vi "ClimbWeightHandler.vi"(8 "error in (no error)":errorcluster, 10 "cClimbWeight":bool, 11 "MainQueue":refnum<queue>) -> (0 "error out":errorcluster)   [LabVIEW 2013]
uses:
  QueueInstruction.ctl
  SubsystemEnum.ctl
  ActionEnum.ctl
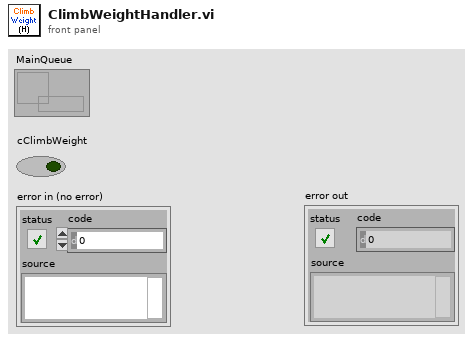
[diagram p1: front panel]
types:
  T1 = typedef "SubsystemEnum.ctl" = enum16{"TankDrive", "FirePneumatic", "Climber", "ClimbWeight", "ShooterAngle"}
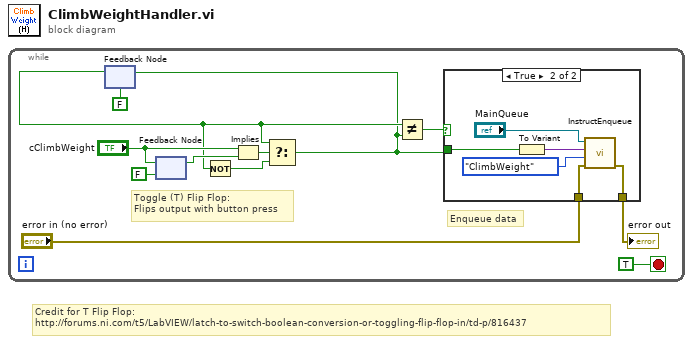
[diagram p0: block diagram]
diagram:
  # "Credit for T Flip Flop:\nhttp://forums.ni.com/t5/LabVIEW/latch-to-switch-boolean-conversion-or-toggling-flip-flop-in/td-p/816437"
  n1 = while {
    stop <- TRUE stop-if-true
    # "Enqueue data"
    # "Toggle (T) Flip Flop:\nFlips output with button press"
    n2 = feedback #1(FALSE) -> (w4:bool)
    n3 = feedback #2(FALSE ("cClimbWeight")) -> (w6:bool)
    n4 = feedback-in #2("cClimbWeight") -> ()
    n5 = Not(x=w4) -> (.not. x?=w9:bool)
    n6 = Implies(1:w6, 2:"cClimbWeight") -> (0:w8:bool)
    n7 = Select(t=w4, s=w8, f=w9) -> (s? t:f=w3:bool)
    n8 = feedback-in #1(w3) -> ()
    n9 = Not Equal?(x=w4, y=w3) -> (x != y?=w5:bool)
    n10 = case shown="True" w5 {
      tunnel: "error in (no error)" -> [w13 w15]
      tunnel: [w13 w14] -> w10
      tunnel: w3 -> [_ w19]
      frame False {
      }
      frame True {
        n11 = To Variant(anything=w19) -> (Variant=w18:variant)
        n12 = call "InstructEnqueue.vi"("error in (no error)"=w15, "Subsystem"=SubsystemEnum."ClimbWeight", "Variant"=w18, "Queue"="MainQueue") -> ("error out"=w14:errorcluster)  [unwired: 7 in]
      }
    }
    "error out" <- w10
  }
